vi "Destroy.vi"(8 "Error In":errorcluster, 11 "reference in":refnum<class "TemplateGUI.lvclass">) -> (0 "Error Out":errorcluster, 3 "reference out":refnum<class "TemplateGUI.lvclass">)   [LabVIEW 2021, in "TemplateGUI.lvlib" / "TemplateGUI.lvclass"]
uses:
  TemplateGUI.lvclass
  .Externals/Library_TAF_ApplicationFramework/TAFBaseGUI/TAFBaseGUI.lvclass
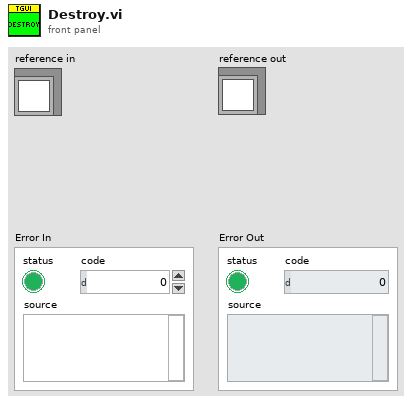
[diagram p1: front panel]
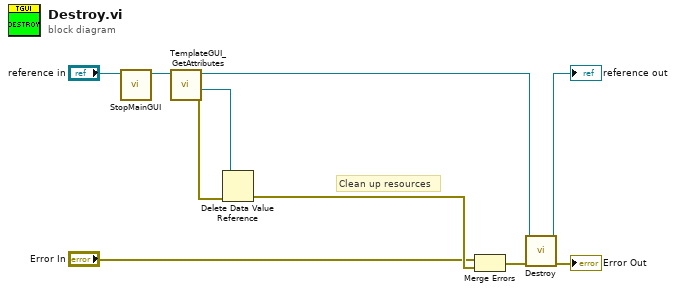
[diagram p0: block diagram]
diagram:
  # "Clean up resources"
  n1 = call "StopMainGUI.vi"("reference in"="reference in") -> ("reference out"=w5:refnum<class "TemplateGUI.lvclass">)  [unwired: 9 in, 1 out]
  n2 = call "TemplateGUI_GetAttributes.vi"("reference in"=w5) -> ("error out"=w10:errorcluster, "DataRef"=w9:refnum<data-value>, "reference out"=w4:refnum<class "TemplateGUI.lvclass">)  [unwired: 7 in, 1 out]
  n3 = Delete Data Value Reference(data value reference=w9, error in=w10) -> (error out=w8:errorcluster)  [unwired: 1 out]
  n4 = Merge Errors("Error In", w8) -> (w2:errorcluster)
  n5 = call-parent "Destroy.vi"("Error In"=w2, "reference in"=w4) -> ("Error Out"=→"Error Out":errorcluster, "reference out"=→"reference out":refnum<class "TemplateGUI.lvclass">)  [unwired: 8 in]
